vi "Fail If Error.vi"(7 "Description":string, 8 "error in (no error)":errorcluster, 10 "Assert error":errorcluster, 11 "LUnit Test Case In":refnum<class "LUnit Test Case.lvclass">) -> (0 "error out":errorcluster, 3 "LUnit Test Case Out":refnum<class "LUnit Test Case.lvclass">)   [LabVIEW 2020, in "LUnit Test Case.lvclass"]
doc: "Generates a fail result for the calling test method if the inputs contains an error with status \"True\". A description may be provided to the result."
uses:
  LUnit Test Case.lvclass
  Result/Type.ctl
  LUnit Test Case.lvclass/LUnit Test Case.ctl
  Private/Run In UI.vi
  <vilib>/Utility/error.llb/Clear Errors.vi
  Result/Result.lvlib
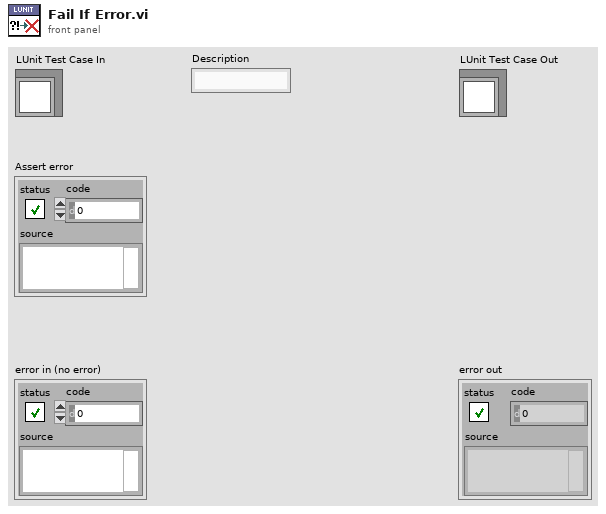
[diagram p1: front panel]
types:
  T1 = typedef "Result.lvlib/Type.ctl" = enum16{"Test Case", "Test Suite", "Test Run", "Pass", "Fail", "Skip", "Pass if", "Fail if", "Pass if Error", "Fail if Error", "Pass if Equal", "Fail if Equal"}
  T2 = cluster{"Expected":variant, "Actual":variant, "Delta":variant}
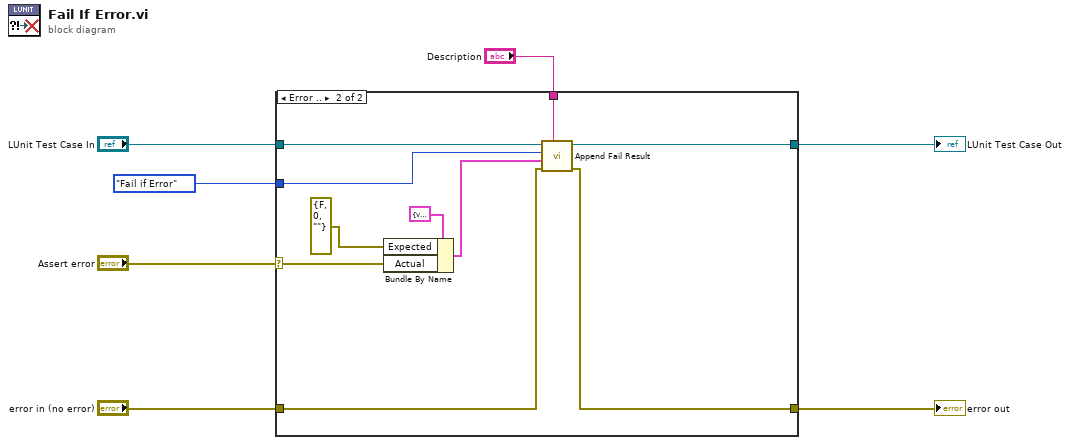
[diagram p0: block diagram]
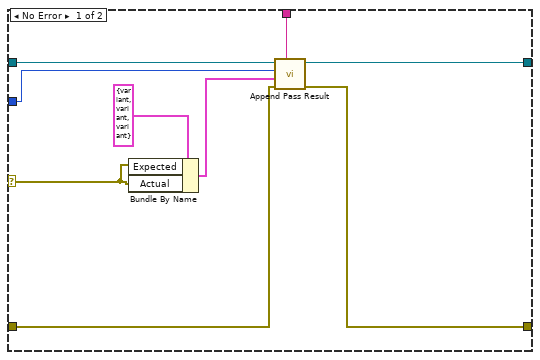
[diagram p2: hidden frame]
diagram:
  n1 = case shown="Error .." "Assert error" {
    selector: "Assert error" -> [w9 w19]
    tunnel: "LUnit Test Case In" -> [w16 w26]
    tunnel: [w15 w25] -> w6
    tunnel: [w14 w24] -> w5
    tunnel: "Description" -> [w13 w23]
    tunnel: "error in (no error)" -> [w12 w22]
    tunnel: Type."Fail if Error" ("Result Type") -> [w11 w21]
    frame No Error {
      n2 = Bundle By Name(cluster=T2 {"Expected"=variant, "Actual"=variant, "Delta"=variant} ("Data"), "Expected"=w9, "Actual"=w9) -> (w8:T2)
      n3 = call "Append Pass Result.vi"("Description"=w13, "error in (no error)"=w12, "Data"=w8, "Result Type"=w11, "LUnit Test Case In"=w16) -> ("error out"=w14:errorcluster, "LUnit Test Case Out"=w15:refnum<class "LUnit Test Case.lvclass">)  [unwired: 5 in]
    }
    frame Error {
      n4 = Bundle By Name(cluster=T2 {"Expected"=variant, "Actual"=variant, "Delta"=variant} ("Data"), "Expected"=errorcluster {"status"=FALSE, "code"=0, "source"=""} ("error IO"), "Actual"=w19) -> (w17:T2)
      n5 = call "Append Fail Result.vi"("Description"=w23, "error in (no error)"=w22, "Data"=w17, "Result Type"=w21, "LUnit Test Case In"=w26) -> ("error out"=w24:errorcluster, "LUnit Test Case Out"=w25:refnum<class "LUnit Test Case.lvclass">)  [unwired: 5 in]
    }
  }
  "error out" <- w5
  "LUnit Test Case Out" <- w6
